vi "Intake Controller.vi"(8 "error in":errorcluster) -> ()   [LabVIEW 2015]
doc: "This VI executes continuously carrying out the current operation and responding to updates or new operations. It will often contain the timing or control code that is difficult to place directly in TeleOp. This VI generally opens all sensors and motors and isolates the rest of the robot code from knowing how the operations are carried out."
uses:
  Intake Setpoints.ctl
  Intake Operations.ctl
  <vilib>/Rock Robotics/SystemInterfaces/DIO/FPGA_DIOPWMChannel.ctl
  <vilib>/Rock Robotics/WPI/SafetyOutput/WPI_SafetyOutputConfigMenu.ctl
  <vilib>/Rock Robotics/WPI/MotorControl/WPI_MotorControlOpen SPARK.vi
  <vilib>/Rock Robotics/WPI/Solenoid/Deprecated/WPI_SolenoidSetBool.vi
  <vilib>/Rock Robotics/Network Tables/NT Write Boolean.vi
panel:
  out "Current\nCmd":string
  # "Tip: It may be helpful to observe inputs and sensor values.\nYou may also want to display tuning or debugging controls."
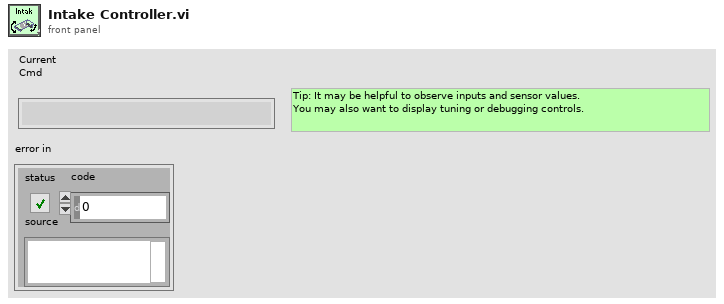
[diagram p1: front panel]
types:
  T1 = typedef "WPI_SafetyOutputConfigMenu.ctl" = enum16{"Enable", "Disable"}
  T2 = typedef "FPGA_DIOPWMChannel.ctl" = enum8{"PWM 0", "PWM 1", "PWM 2", "PWM 3", "PWM 4", "PWM 5", "PWM 6", "PWM 7", "PWM 8", "PWM 9", "PWM MXP 0", "PWM MXP 1", "PWM MXP 2", "PWM MXP 3", "PWM MXP 4", "PWM MXP 5", "PWM MXP 6", "PWM MXP 7", "PWM MXP 8", "PWM MXP 9", "Invalid"}
  T3 = typedef "Intake Setpoints.ctl" = cluster{"Operation":T4, "Setpoint":dbl, "Duration":dbl, "OnOff":bool}
  T4 = typedef "Intake Operations.ctl" = enum16{"Reserve", "Read Current", "Immediate", "Move Arm", "ManualIntake", "AutoIntake"}
  T5 = typedef "WPI_MotorControlDeviceRef.ctl" = cluster{"DeviceStatus":errorcluster, "Type":T6, "PWM":cluster{"PWM Channel":T2, "DeadBand":T7}, "CAN":cluster{"Device Number":u8, "Control Mode":T8, "Semaphore":T9, "Max Vout":dbl, "TalonSRX Control Mode":T10}, "Invert":bool}
  T6 = typedef "WPI_MotorControlType.ctl" = enum16{"PWM", "CAN", "CANTalonSRX"}
  T7 = typedef "WPI_PWMDeadband.ctl" = cluster{"Name":string, "maxPositivePwm":i32, "minPositivePwm":i32, "centerPwm":i32, "maxNegativePwm":i32, "minNegativePwm":i32, "angularRange":u16}
  T8 = typedef "WPI_CANJaguar_ControlMode.ctl" = enum8{"Percent VBus", "Current", "Speed", "Position", "Voltage"}
  T9 = typedef "Semaphore RefNum" = refnum<k1>
  T10 = typedef "WPI_CANTalonSRX_APIControlMode.ctl" = enum8{"Percent VBus", "Speed", "Position", "Slave", "Unchanged / Invalid", "Voltage Compensation", "Current", "Motion Profile"}
  T11 = typedef "WPI_SolenoidDevRef.ctl" = cluster{"DevStatus":errorcluster, "Pneumatics Control Module":u8, "Forward Solenoid Channel":T12, "Reverse Solenoid Channel":T12}
  T12 = typedef "WPI_SolenoidChannel.ctl" = enum8{"Solenoid 0", "Solenoid 1", "Solenoid 2", "Solenoid 3", "Solenoid 4", "Solenoid 5", "Solenoid 6", "Solenoid 7", "Invalid"}
  T13 = typedef "Command Status Info.ctl" = cluster{"Name":string, "Status":T14, "notifier out":T15}
  T14 = typedef "Completion Status.ctl" = enum16{"Successful", "Aborted", "Incomplete"}
  T15 = typedef "Completion Notifier.ctl" = refnum<notifier>
  T16 = cluster{"Default Command":T3, "Command Timing":cluster{"Start Time (ms)":u32, "Iterations":i32}, "Command Arguments":cluster{"Command Info":T13, "Description":string, "Default Command":T3, "notifier out":refnum<notifier>, "Subsystem Name":string}}
  T17 = typedef "WPI_SwitchDevRef.ctl" = cluster{"DevStatus":errorcluster, "DIO Channel":T18, "CntIndex":T19, "Normally Closed":bool}
  T18 = typedef "FPGA_DIOChannel.ctl" = enum8{"DIO 0", "DIO 1", "DIO 2", "DIO 3", "DIO 4", "DIO 5", "DIO 6", "DIO 7", "DIO 8", "DIO 9", "DIO MXP 0", "DIO MXP 1", "DIO MXP 2", "DIO MXP 3", "DIO MXP 4", "DIO MXP 5", "DIO MXP 6", "DIO MXP 7", "DIO MXP 8", "DIO MXP 9", "DIO MXP 10", "DIO MXP 11", "DIO MXP 12", "DIO MXP 13", "DIO MXP 14", "DIO MXP 15", "Invalid"}
  T19 = typedef "FPGA_CounterCtrSystemIndex.ctl" = enum8{"Ctr 0", "Ctr 1", "Ctr 2", "Ctr 3", "Ctr 4", "Ctr 5", "Ctr 6", "Ctr 7", "Invalid"}
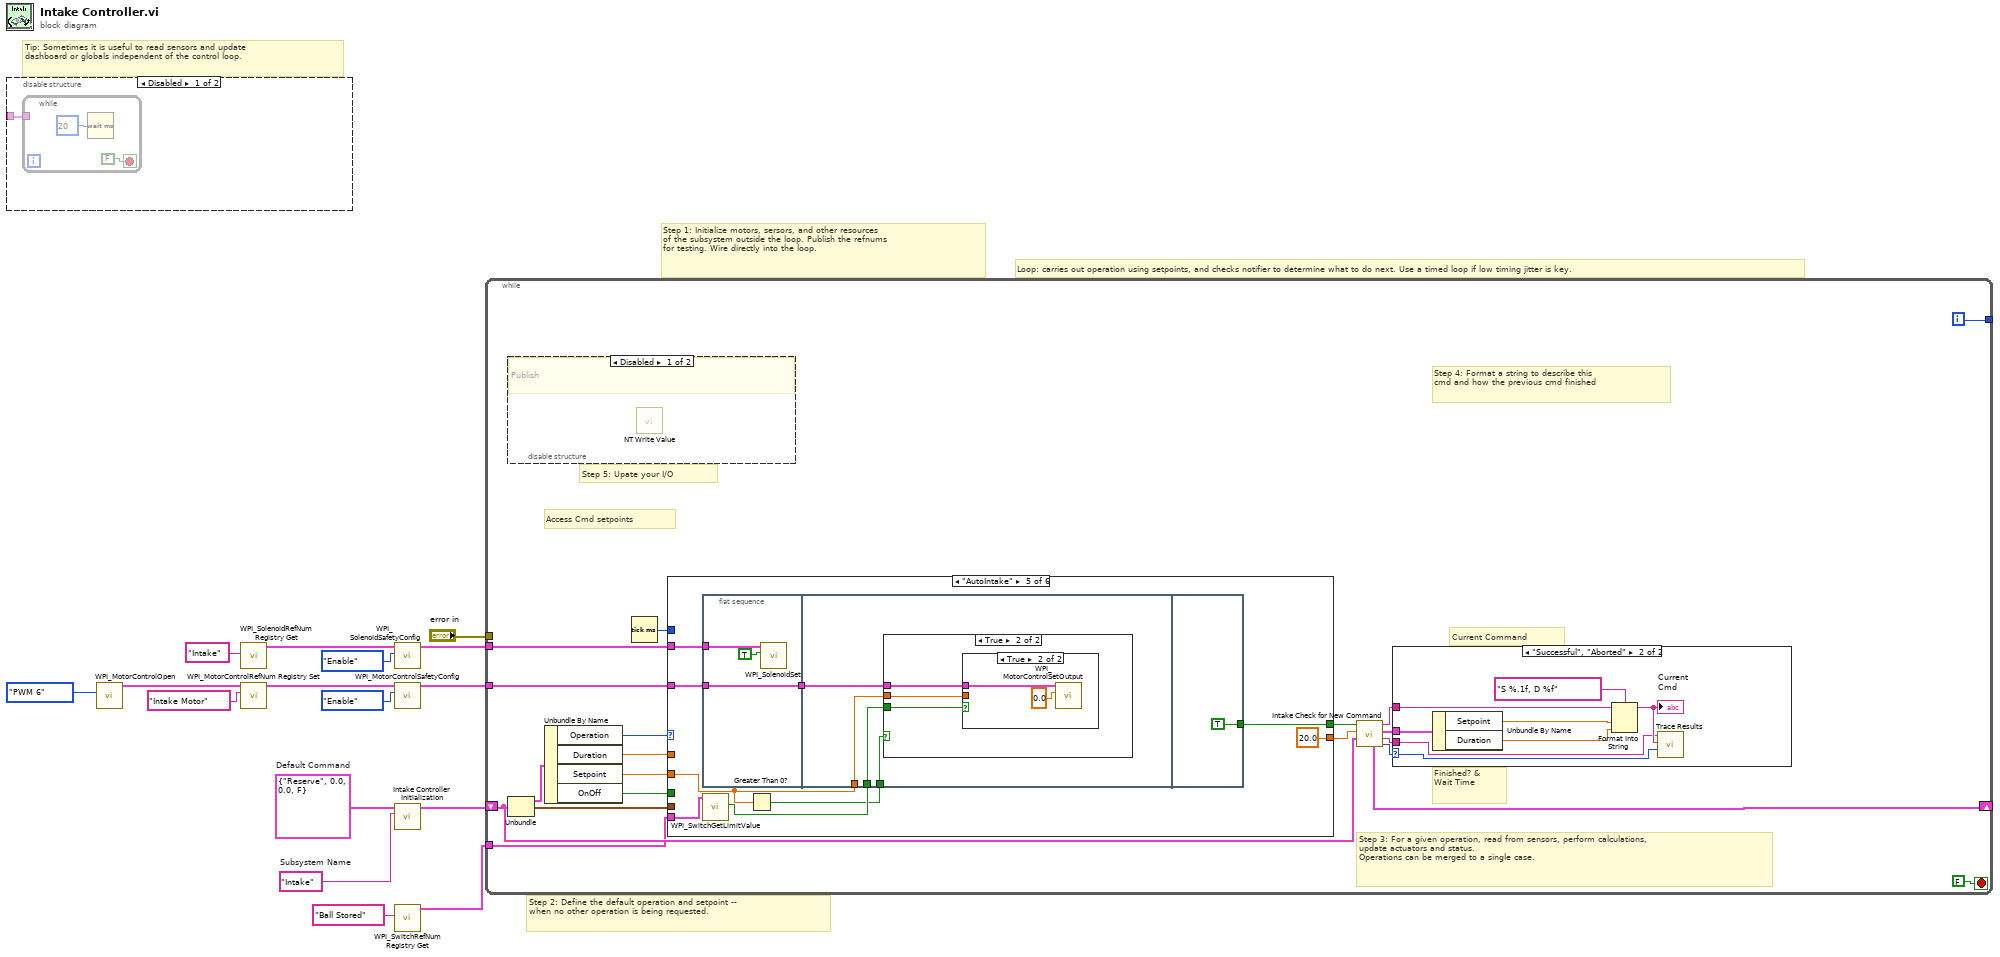
[diagram p0: block diagram]
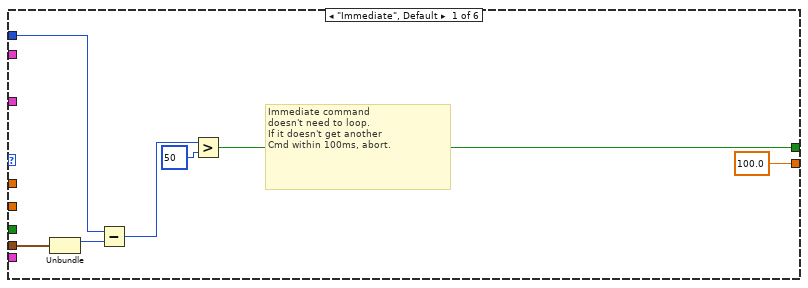
[diagram p3: hidden frame]
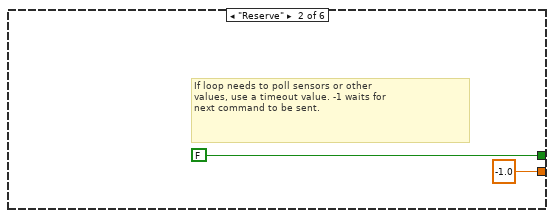
[diagram p4: hidden frame]
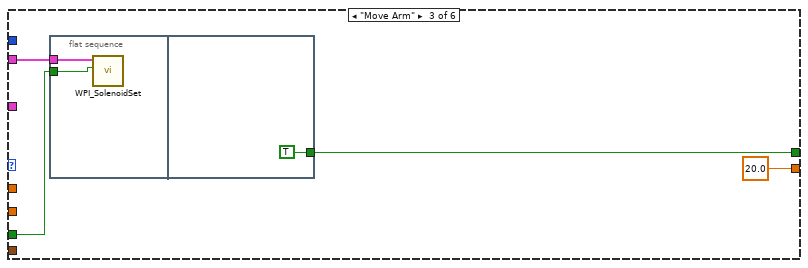
[diagram p5: hidden frame]
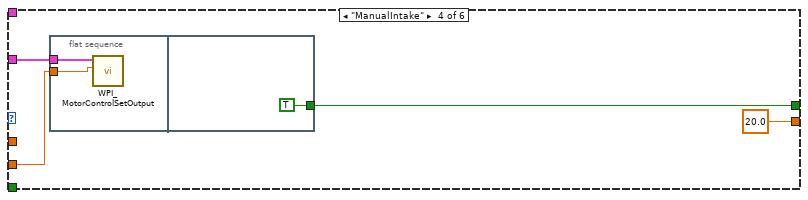
[diagram p6: hidden frame]
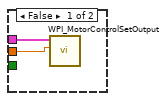
[diagram p7: hidden frame]
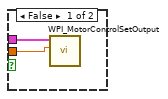
[diagram p8: hidden frame]
diagram:
  w13 = T3 {"Operation"=enum."Reserve", "Setpoint"=0.0, "Duration"=0.0, "OnOff"=FALSE}  # Default Command
  w14 = "Intake"  # Subsystem Name
  # "Tip: Sometimes it is useful to read sensors and update\ndashboard or globals independent of the control loop."
  # "Step 2: Define the default operation and setpoint --\nwhen no other operation is being requested."
  # "Step 1: Initialize motors, sersors, and other resources\nof the subsystem outside the loop. Publish the refnums\nfor testing. Wire directly into the loop."
  # "Loop: carries out operation using setpoints, and checks notifier to determine what to do next. Use a timed loop if low timing jitter is key."
  n1 = disable-structure shown="Disabled" {
    disable-tunnel: _ -> [w17 _]
    frame Disabled {
      n2 = while {
        tunnel: w17 -> [_]
        stop <- FALSE stop-if-true
        n3 = Wait (ms)(milliseconds to wait=u32 20) -> ()  [unwired: 1 out]
      }
    }
    frame Enabled {
    }
  }
  n4 = call-poly <vilib>:"WPI_MotorControlOpen.vi"("PWM Channel"=FPGA_DIOPWMChannel."PWM 6") -> ("MotorControlDeviceRef"=w12:T5)  [unwired: 9 in, 1 out]
  n5 = call <vilib>:"WPI_SolenoidRefNum Registry Get.vi"("refnum name"="Intake") -> ("SolenoidDevRef"=w6:T11)  [unwired: 9 in, 1 out]
  n6 = call <vilib>:"WPI_MotorControlRefNum Registry Set.vi"("refnum name"="Intake Motor", "MotorControlDevRef"=w12) -> ("MotorControlDevRef"=w11:T5)  [unwired: 8 in, 1 out]
  n7 = call <vilib>:"WPI_SolenoidSafetyConfig.vi"("mode"=WPI_SafetyOutputConfigMenu."Enable", "SolenoidDevRef"=w6) -> ("SolenoidDevRef"=w3:T11)  [unwired: 8 in, 1 out]
  n8 = call <vilib>:"WPI_MotorControlSafetyConfig.vi"("mode"=WPI_SafetyOutputConfigMenu."Enable", "MotorControlDevRef"=w11) -> ("MotorControlDevRef"=w10:T5)  [unwired: 8 in, 1 out]
  n9 = call "Intake Controller Initialization.vi"("Subsystem Name"=w14, "Default Command"=w13) -> ("Command Info"=w15:T16)  [unwired: 9 in]
  n10 = call <vilib>:"WPI_SwitchRefNum Registry Get.vi"("refnum name"="Ball Stored") -> ("SwitchDevRef"=w1:T17)  [unwired: 9 in, 1 out]
  n11 = while {
    shift-right: [w30] -> _
    shift-left: w15 -> [w31]
    tunnel: [w38] -> _
    tunnel: "error in" -> [_]
    tunnel: w10 -> [w23]
    tunnel: w3 -> [w22]
    tunnel: w1 -> [w20]
    i -> [w38]
    stop <- FALSE stop-if-true
    # "Step 5: Upate your I/O"
    # "Step 4: Format a string to describe this\ncmd and how the previous cmd finished"
    # "Current Command"
    # "Access Cmd setpoints"
    # "Finished? &\nWait Time"
    # "Step 3: For a given operation, read from sensors, perform calculations,\nupdate actuators and status.\nOperations can be merged to a single case."
    n12 = disable-structure shown="Disabled" {
      frame Disabled {
        # "Publish"
        n13 = call-poly <vilib>:"NT Write Value.vi"() -> ()  [unwired: 11 in, 1 out]
      }
      frame Enabled {
      }
    }
    n14 = Unbundle(w31) -> ("Default Command"=w37:T3, "Command Timing"=w33:cluster{"Start Time (ms)":u32, "Iterations":i32})  [unwired: 1 out]
    n15 = Unbundle By Name(w37) -> ("Operation"=w36:T4, "Duration"=w35:dbl, "Setpoint"=w32:dbl, "OnOff"=w21:bool)
    n16 = Tick Count (ms)() -> (millisecond timer value=w34:u32)
    n17 = case shown="\"AutoIntake\"" w36 {
      tunnel: [100.0 -1.0 20.0 20.0 20.0 _] -> w28
      tunnel: [w40 FALSE ("ignore previous (F)") w51 w56 w71 _] -> w29
      tunnel: w33 -> [w42 _ _ _ _ _]
      tunnel: w35 -> [_ _ _ _ _ _]
      tunnel: w34 -> [w41 _ _ _ _ _]
      tunnel: w32 -> [_ _ _ w58 w65 _]
      tunnel: w23 -> [_ _ _ w59 w70 _]
      tunnel: w22 -> [_ _ w50 _ w67 _]
      tunnel: w21 -> [_ _ w49 _ _ _]
      tunnel: w20 -> [_ _ _ _ w69 _]
      frame "Immediate", Default {
        # "Immediate command\ndoesn't need to loop.\nIf it doesn't get another\nCmd within 100ms, abort."
        n18 = Unbundle(w42) -> ("Start Time (ms)"=w45:u32)  [unwired: 1 out]
        n19 = Subtract(x=w41, y=w45) -> (x-y=w44:u32)
        n20 = Greater?(x=w44, y=u8 50 ("Left Motor")) -> (0:w40:bool)
      }
      frame "Reserve" {
        # "If loop needs to poll sensors or other\nvalues, use a timeout value. -1 waits for\nnext command to be sent."
      }
      frame "Move Arm" {
        n21 = flat-sequence {
          tunnel: w50 -> [w54]
          tunnel: w49 -> [w53]
          tunnel: [TRUE] -> w51
          frame #0 {
            n22 = call-poly <vilib>:"WPI_SolenoidSet.vi"("Value"=w53, "SolenoidDevRef"=w54) -> ()  [unwired: 8 in, 2 out]
          }
          frame #1 {
          }
        }
      }
      frame "ManualIntake" {
        n23 = flat-sequence {
          tunnel: w59 -> [w61]
          tunnel: w58 -> [w60]
          tunnel: [TRUE] -> w56
          frame #0 {
            n24 = call <vilib>:"WPI_MotorControlSetOutput.vi"("Output"=w60, "MotorControlDevRef"=w61) -> ()  [unwired: 7 in, 3 out]
          }
          frame #1 {
          }
        }
      }
      frame "AutoIntake" {
        n25 = flat-sequence {
          tunnel: w70 -> [w74]
          tunnel: [w74] -> w68
          tunnel: w67 -> [w73]
          tunnel: w65 -> [w77]
          tunnel: w68 -> [w78]
          tunnel: w66 -> [w76]
          tunnel: w64 -> [w75]
          tunnel: [TRUE] -> w71
          frame #0 {
            n26 = call-poly <vilib>:"WPI_SolenoidSet.vi"("Value"=TRUE, "SolenoidDevRef"=w73) -> ()  [unwired: 8 in, 2 out]
          }
          frame #1 {
            n27 = case shown="True" w75 {
              tunnel: w78 -> [w80 w83]
              tunnel: w77 -> [w79 w82]
              tunnel: w76 -> [_ w81]
              frame False {
                n28 = call <vilib>:"WPI_MotorControlSetOutput.vi"("Output"=w79, "MotorControlDevRef"=w80) -> ()  [unwired: 7 in, 3 out]
              }
              frame True {
                n29 = case shown="True" w81 {
                  tunnel: w83 -> [w84 w87]
                  tunnel: w82 -> [w85 _]
                  frame False {
                    n30 = call <vilib>:"WPI_MotorControlSetOutput.vi"("Output"=w85, "MotorControlDevRef"=w84) -> ()  [unwired: 7 in, 3 out]
                  }
                  frame True {
                    n31 = call <vilib>:"WPI_MotorControlSetOutput.vi"("Output"=0.0, "MotorControlDevRef"=w87) -> ()  [unwired: 7 in, 3 out]
                  }
                }
              }
            }
          }
          frame #2 {
          }
        }
        n32 = call <vilib>:"WPI_SwitchGetLimitValue.vi"("SwitchDevRef"=w69) -> ("Switch Pressed"=w66:bool)  [unwired: 8 in, 2 out]
        n33 = Greater Than 0?(x=w65) -> (x > 0?=w64:bool)
      }
      frame "Read Current" {
      }
    }
    n34 = call "Intake Check for New Command.vi"("Current Command"=w31, "Wait time (ms)"=w28, "Finished?"=w29) -> ("Completion"=w24:T14, "Subsystem Name"=w25:string, "Current Command"=w26:T3, "Initial Trace String"=w27:string, "NextCommand"=w30:T16)  [unwired: 4 in]
    n35 = case shown="\"Successful\", \"Aborted\"" w24 {
      selector: w24 -> [_ w96]
      tunnel: w27 -> [_ w92]
      tunnel: w26 -> [_ w93]
      tunnel: w25 -> [_ w89]
      frame "Incomplete", Default {
        # "Continuing current command"
      }
      frame "Successful", "Aborted" {
        # "Report and setup for next command"
        n36 = Unbundle By Name(w93) -> ("Setpoint"=w95:dbl, "Duration"=w90:dbl)
        n37 = Format Into String(format string="S %.1f, D %f", initial string=w92, w95, w90) -> (resulting string=w91:string)  [unwired: 1 in, 1 out]
        "Current\nCmd" <- w91
        n38 = call <vilib>:"Trace Results.vi"("Status of previous command"=w96, "Description"=w91, "Subsystem"=w89) -> ()  [unwired: 9 in]
      }
    }
  }
